vi "Run Transient Capture Demonstration.vi"() -> ()   [LabVIEW 2017]
doc: "Run a demonstration using a device driver, with the data shared across a local network.\n\nUses a configurable GUI, with multiple tabs and active plots."
uses:
  GUI/Plots/Plot Data - Main GUI.vi
  GUI/Plots/DTacq Plot Display Library.lvlib
  DTACQ - Network Enabled Device Driver.lvlib
panel:
  in  "Maximum Waveforms per Second":dbl=1000.0
  in  "Soft Trigger":bool
  in  "Start Button":bool
  in  "Waveform Length (Samples)":i32=1000
  in  "Configuration file path (Leave Blank for Defaults)":path
  # "Transient Capture"
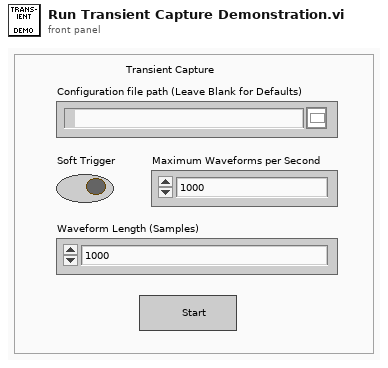
[diagram p1: front panel]
types:
  T1 = enum32{"Invalid", "Standard", "Closed", "Hidden", "Minimized", "Maximized"}
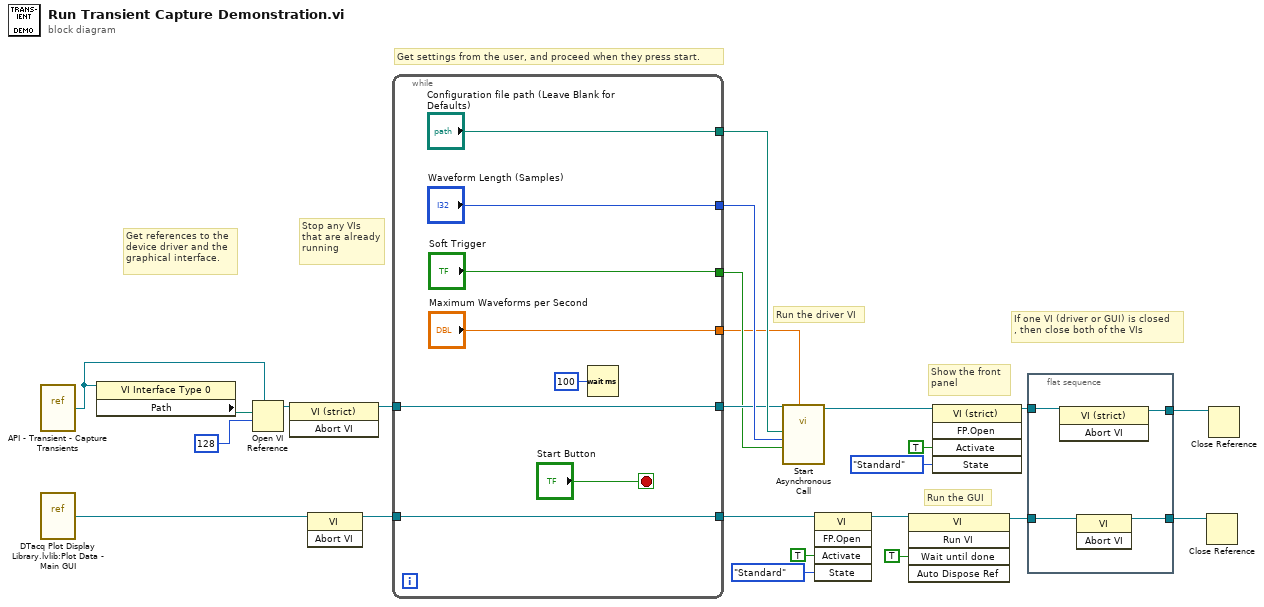
[diagram p0: block diagram]
diagram:
  # "Show the front\npanel"
  # "If one VI (driver or GUI) is closed\n, then close both of the VIs"
  # "Run the GUI"
  # "Run the driver VI"
  # "Get settings from the user, and proceed when they press start."
  # "Stop any VIs\nthat are already\nrunning"
  # "Get references to the\ndevice driver and the\ngraphical interface."
  n1 = vi-ref "API - Transient - Capture Transients.vi"() -> (w7:refnum<vi>)
  n2 = vi-ref "DTacq Plot Display Library.lvlib:Plot Data - Main GUI.vi"() -> (w22:refnum<vi>)
  n3 = property class="VI Interface Type 0"(reference=w7) -> ("Path"=w8:path)  [unwired: 1 in, 2 out]
  n4 = Open VI Reference(type specifier VI Refnum (for type only)=w7, vi path=w8, options=128) -> (vi reference=w5:refnum<vi>)  [unwired: 3 in, 1 out]
  n5 = invoke class="VI (strict)" method="Abort VI"(reference=w5) -> (reference out=w14:refnum<vi>)  [unwired: 2 in, 2 out]
  n6 = invoke class="VI" method="Abort VI"(reference=w22) -> (reference out=w12:refnum<vi>)  [unwired: 2 in, 2 out]
  n7 = while {
    tunnel: ["Configuration file path (Leave Blank for Defaults)"] -> w16
    tunnel: ["Waveform Length (Samples)"] -> w15
    tunnel: w14 -> [w30]
    tunnel: [w30] -> w13
    tunnel: w12 -> [w29]
    tunnel: [w29] -> w11
    tunnel: ["Soft Trigger"] -> w10
    tunnel: ["Maximum Waveforms per Second"] -> w9
    stop <- "Start Button" stop-if-true
    n8 = Wait (ms)(milliseconds to wait=u32 100) -> ()  [unwired: 1 out]
  }
  n9 = call-by-ref "Start Asynchronous Call"(reference=w13, "Maximum Waveforms/Second"=w9, "Soft Trigger"=w10, "Maximum Waveform Length"=w15, "configuration file path"=w16) -> (reference out=w4:refnum<vi>)  [unwired: 8 in, 2 out]
  n10 = invoke class="VI" method="FP.Open"(reference=w11, "Activate"=TRUE ("Activate?"), "State"=T1."Standard") -> (reference out=w21:refnum<vi>)  [unwired: 2 in, 4 out]
  n11 = invoke class="VI" method="Run VI"(reference=w21, "Wait until done"=TRUE ("Wait Until Done")) -> (reference out=w19:refnum<vi>)  [unwired: 3 in, 4 out]
  n12 = invoke class="VI (strict)" method="FP.Open"(reference=w4, "Activate"=TRUE ("Activate?"), "State"=T1."Standard") -> (reference out=w3:refnum<vi>)  [unwired: 2 in, 4 out]
  n13 = flat-sequence {
    tunnel: w3 -> [w36]
    tunnel: w19 -> [w35]
    tunnel: [w34] -> w18
    tunnel: [w33] -> w17
    frame #0 {
      n14 = invoke class="VI (strict)" method="Abort VI"(reference=w36) -> (reference out=w33:refnum<vi>)  [unwired: 2 in, 2 out]
      n15 = invoke class="VI" method="Abort VI"(reference=w35) -> (reference out=w34:refnum<vi>)  [unwired: 2 in, 2 out]
    }
  }
  n16 = Close Reference(reference=w18) -> ()  [unwired: 1 in, 1 out]
  n17 = Close Reference(reference=w17) -> ()  [unwired: 1 in, 1 out]
